vi "AddLogEntry.vi"(8 "error in (no error)":errorcluster, 11 "VISA Refnum in":refnum<visa-resource-name>) -> (0 "error out":errorcluster, 3 "VISA Refnum out":refnum<visa-resource-name>)   [LabVIEW 2023, in "BigSkyControl.lvlib"]
uses:
  BigSkyControl.lvlib
panel:
  out "log entry string":string
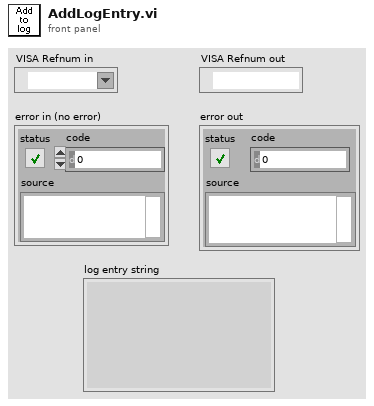
[diagram p1: front panel]
types:
  T1 = enum16{"open", "replace", "create", "open or create", "replace or create", "replace or create with confirmation"}
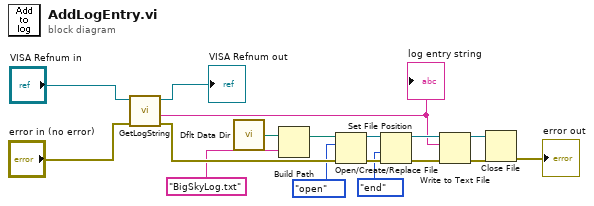
[diagram p0: block diagram]
diagram:
  n1 = call "GetLogString.vi"("error"="error in (no error)", "VISA resource"="VISA Refnum in") -> ("error out"=w11:errorcluster, "log entry string"=w12:string, "VISA resource out"=→"VISA Refnum out":refnum<visa-resource-name>)  [unwired: 7 in]
  "log entry string" <- w12
  n2 = call <vilib>:"Dflt Data Dir.vi"() -> ("App:Default Data Directory"=w2:path)
  n3 = Build Path(base path=w2, name or relative path="BigSkyLog.txt") -> (appended path=w4:path)
  n4 = Open/Create/Replace File(file path (use dialog)=w4, error in=w11, operation (0:open)=T1."open") -> (refnum out=w9:refnum<file>, error out=w10:errorcluster)  [unwired: 3 in, 1 out]
  n5 = Set File Position(refnum=w9, from (0:start)=enum16{"start", "end", "current"}."end", error in=w10) -> (refnum out=w13:refnum<file>, error out=w14:errorcluster)  [unwired: 1 in]
  n6 = Write to Text File(file (use dialog)=w13, text=w12, error in=w14) -> (refnum out=w16:refnum<file>, error out=w15:errorcluster)  [unwired: 1 in, 1 out]
  n7 = Close File(refnum=w16, error in=w15) -> (error out=→"error out":errorcluster)  [unwired: 1 out]
